vi "TemperatureAlarm.vi"() -> ()   [LabVIEW 2020]
doc: "This VI connects to the Arduino, receives the temperature and displays it on the graph. By temperature and the threshold values controls RGB diode."
uses:
  <vilib>/Instr/_visa.llb/VISA Flush IO Buffer Mask.ctl
  <vilib>/Instr/_visa.llb/VISA Configure Serial Port (Instr).vi
panel:
  in  "T_L":u32(colorbox)=16860 caption="Temperatura poniżej progu"
  in  "T_V":dbl=10.0 caption="Próg temperatury [°C]" format="%#_4g"
  out "Chart":dbl(graph)
  in  "VISA resource name":refnum<visa-resource-name>="COM7" caption="Port"
  in  "T_H":u32(colorbox)=16711680 caption="Temperatura powyżej progu"
  in  "stop":bool
  # "Ustawienia LED"
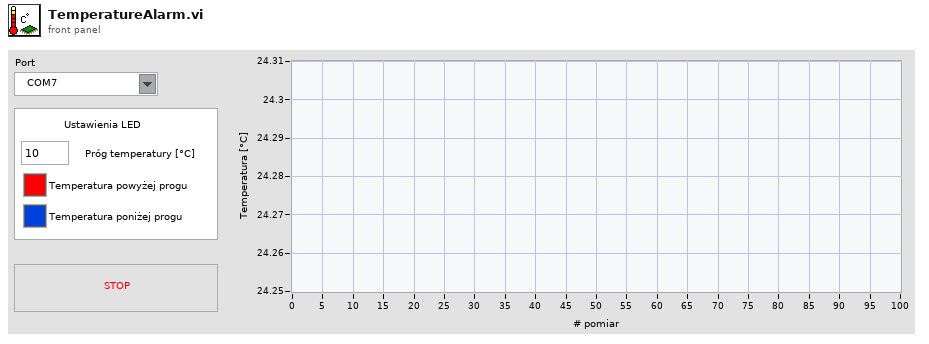
[diagram p1: front panel]
types:
  T1 = typedef "VISA Flush IO Buffer Mask.ctl" = u16
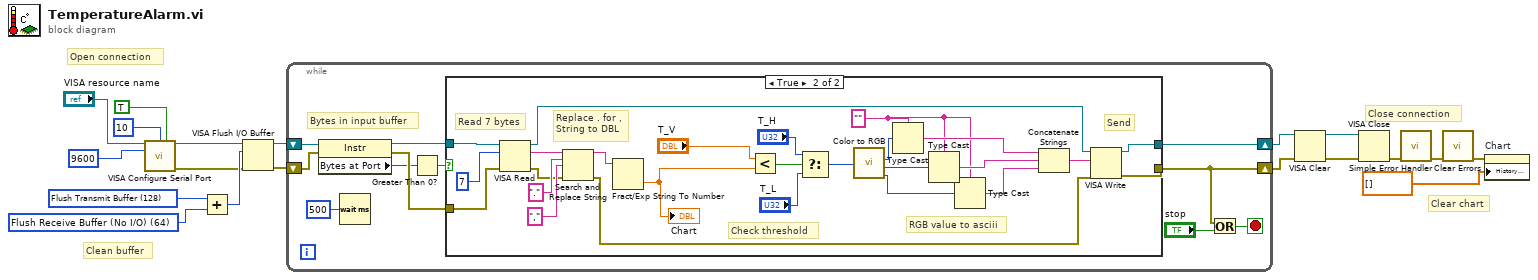
[diagram p0: block diagram]
diagram:
  w8 = T1 64 items=["Flush Receive Buffer"=16, "Write Transmit Buffer to Device"=32, "Flush Receive Buffer (No I/O)"=64, "Flush Transmit Buffer"=128] ("y")
  w10 = T1 128 items=["Flush Receive Buffer"=16, "Write Transmit Buffer to Device"=32, "Flush Receive Buffer (No I/O)"=64, "Flush Transmit Buffer"=128] ("Mask")
  # "Clean buffer"
  # "Clear chart"
  # "Open connection"
  # "Close connection"
  n1 = call-poly "VISA Configure Serial Port"("VISA resource name"="VISA resource name", "termination char\n(0xA = '\\n' = LF)"=u8 10 ("termination char\n(0xA = '\\n' = LF)"), "Enable Termination\nChar (T)"=TRUE ("Enable Termination\nChar (T)"), "baud rate (9600)"=u32 9600) -> ("VISA resource name out"=w5:refnum<visa-resource-name>, "error out"=w7:errorcluster)  [unwired: 10 in]
  n2 = Add(x=w10, y=w8) -> (x+y=w9:T1)
  n3 = VISA Flush I/O Buffer(VISA resource name=w5, mask (16)=w9, error in (no error)=w7) -> (VISA resource name out=w4:refnum<visa-resource-name>, error out=w6:errorcluster)
  n4 = while {
    shift-right: [w23] -> w2
    shift-left: w4 -> [w30]
    shift-right: [w21] -> w18
    shift-left: w6 -> [w29]
    stop <- w22 stop-if-true
    # "Bytes in input buffer"
    n5 = property class="Instr"(reference=w30, error in=w29) -> (reference out=w25:refnum<visa-resource-name>, error out=w24:errorcluster, "Bytes at Port"=w20:u32)
    n6 = Wait (ms)(milliseconds to wait=u32 500) -> ()  [unwired: 1 out]
    n7 = Greater Than 0?(x=w20) -> (x > 0?=w26:bool)
    n8 = case shown="True" w26 {
      tunnel: w25 -> [w32 w58]
      tunnel: w24 -> [w31 w57]
      tunnel: [w32 w35] -> w23
      tunnel: [w31 w36] -> w21
      frame False {
      }
      frame True {
        w33 = "" ("format string")
        # "RGB value to asciii"
        # "Send"
        # "Read 7 bytes"
        # "Check threshold"
        # "Replace . for ,\nString to DBL"
        n9 = VISA Read(VISA resource name=w58, byte count=u32 7, error in (no error)=w57) -> (VISA resource name out=w39:refnum<visa-resource-name>, read buffer=w56:string, error out=w38:errorcluster)  [unwired: 1 out]
        n10 = Search and Replace String(input string=w56, search string=".", replace string="," ("replace string (\"\")"), error in=w38) -> (result string=w55:string, error out=w37:errorcluster)  [unwired: 4 in, 2 out]
        n11 = Fract/Exp String To Number(string=w55) -> (number=w51:dbl)  [unwired: 3 in, 1 out]
        "Chart" <- w51
        n12 = Less?(x="T_V", y=w51) -> (x < y?=w50:bool)
        n13 = Select(t="T_H", s=w50, f="T_L") -> (s? t:f=w47:u32)
        n14 = call <vilib>:"Color to RGB.vi"("Color"=w47) -> ("R"=w46:u8, "G"=w45:u8, "B"=w44:u8)  [unwired: 1 out]
        n15 = Type Cast(type=w33, x=w46) -> (*(type *) &x=w41:string)
        n16 = Type Cast(type=w33, x=w45) -> (*(type *) &x=w42:string)
        n17 = Type Cast(type=w33, x=w44) -> (*(type *) &x=w43:string)
        n18 = Concatenate Strings(w41, w42, w43) -> (w40:string)
        n19 = VISA Write(VISA resource name=w39, write buffer=w40, error in (no error)=w37) -> (VISA resource name out=w35:refnum<visa-resource-name>, error out=w36:errorcluster)  [unwired: 1 out]
      }
    }
    n20 = Or(x=w21, y="stop") -> (x .or. y?=w22:bool)
  }
  n21 = VISA Clear(VISA resource name=w2, error in (no error)=w18) -> (VISA resource name out=w1:refnum<visa-resource-name>, error out=w3:errorcluster)
  n22 = VISA Close(VISA resource name=w1, error in (no error)=w3) -> (error out=w17:errorcluster)
  n23 = call <vilib>:"Simple Error Handler.vi"("error in (no error)"=w17) -> ("error out"=w14:errorcluster)  [unwired: 4 in, 4 out]
  n24 = call <vilib>:"Clear Errors.vi"("error in (no error)"=w14) -> ("error out"=w13:errorcluster)  [unwired: 5 in, 1 out]
  n25 = property on="Chart" class="WFChart (strict)"(error in=w13, "History Data"=dbl[] []) -> ()  [unwired: 1 in, 2 out]
